vi "VisionTest.vi"() -> ()   [LabVIEW 2017, in "VisionHW.lvlib"]
uses:
  VisionHW.lvlib
  TypeDefs/ENUM_Vision_Commands.ctl
panel:
  out "concatenated string":string
  in  "Vision_Modes":T1=enum."ResetCamera"
  in  "stop":bool
  in  "VISA Refnum in":refnum<visa-resource-name>
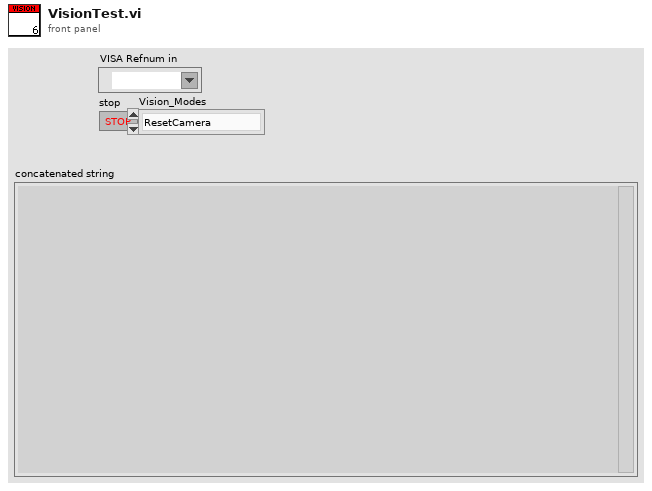
[diagram p1: front panel]
types:
  T1 = typedef "ENUM_Vision_Commands.ctl" = enum16{"Init", "NoOp", "ResetCamera", "VideoOn", "VideoOff", "CubeDetection", "RoadNavigation"}
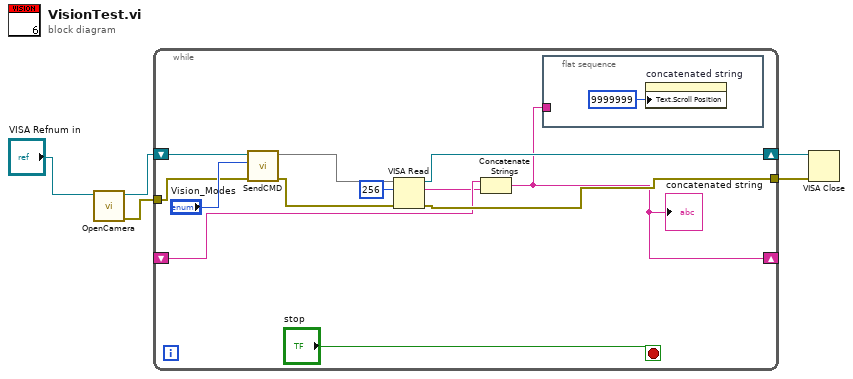
[diagram p0: block diagram]
diagram:
  n1 = call "OpenCamera.vi"("VISA Refnum in"="VISA Refnum in") -> ("error out"=w2:errorcluster, "VISA Refnum out"=w3:refnum<visa-resource-name>)  [unwired: 9 in]
  n2 = while {
    shift-right: [w12] -> w5
    shift-left: w3 -> [w17]
    shift-right: [w6] -> _
    shift-left: _ -> [w8]
    tunnel: w2 -> [w11]
    tunnel: [w9] -> w1
    stop <- "stop" stop-if-true
    n3 = call "SendCMD.vi"("error in (no error)"=w11, "Vision_Modes"="Vision_Modes", 11:w17) -> ("error out"=w10:errorcluster, 3:w13)  [unwired: 7 in]
    n4 = VISA Read(VISA resource name=w13, byte count=u32 256, error in (no error)=w10) -> (VISA resource name out=w12:refnum<visa-resource-name>, read buffer=w7:string, error out=w9:errorcluster)  [unwired: 1 out]
    n5 = Concatenate Strings(w8, w7) -> (w6:string)
    "concatenated string" <- w6
    n6 = flat-sequence {
      tunnel: w6 -> [_]
      frame #0 {
        n7 = property on="concatenated string" class="Str"("Text.Scroll Position"=u32 9999999) -> ()  [unwired: 2 in, 2 out]
      }
    }
  }
  n8 = VISA Close(VISA resource name=w5, error in (no error)=w1) -> ()  [unwired: 1 out]
